vi "Load Config Application.vi"(8 "error In":errorcluster) -> (0 "error Out":errorcluster, 3 "Application Configuration":T1)   [LabVIEW 2021, in "Configuration.lvlib"]
uses:
  Configuration.lvlib
  Typedefs/Application Configuration.ctl
  Module Template/Typedefs/Config.ctl
  Module Template/Module Template.lvlib
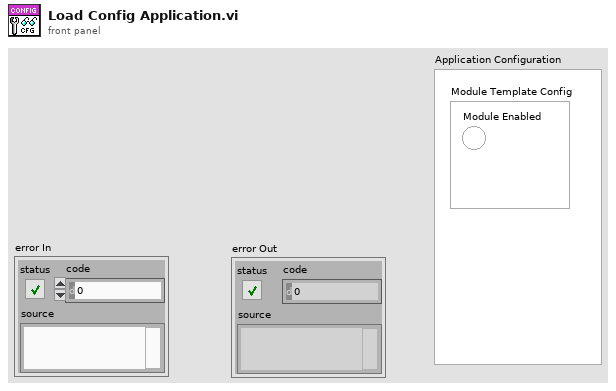
[diagram p1: front panel]
types:
  T1 = typedef "Configuration.lvlib/Application Configuration.ctl" = cluster{"Module Template Config":T2}
  T2 = typedef "Module Template.lvlib/Config.ctl" = cluster{"Module Enabled":bool}
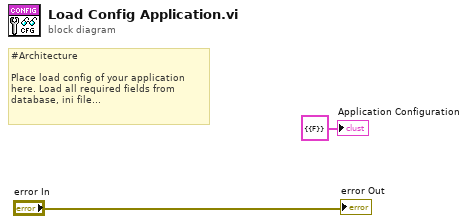
[diagram p0: block diagram]
diagram:
  # "#Architecture\n\nPlace load config of your application \nhere. Load all required fields from \ndatabase, ini file..."
  "Application Configuration" <- T1 {"Module Template Config"={"Module Enabled"=FALSE}} ("Application Configuration")
  "error Out" <- "error In"
